vi "SetPeddleRate.vi"(8 "error in (no error)":errorcluster, 10 "peddle rate":dbl, 11 "Bike in":refnum<class "Bike.lvclass">) -> (0 "error out":errorcluster, 3 "Bike out":refnum<class "Bike.lvclass">)   [LabVIEW 2019, in "Bike.lvclass"]
uses:
  Bike.lvclass
  Bike.lvclass/Bike.ctl
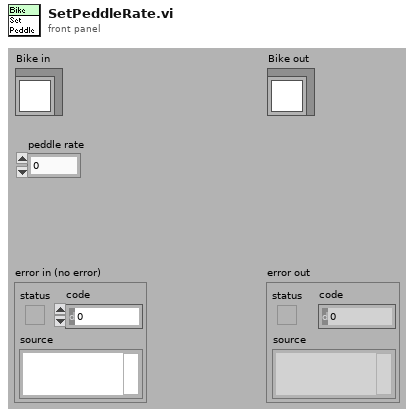
[diagram p1: front panel]
types:
  T1 = typedef "Bike.lvclass/DataRef.ctl" = refnum<data-value>
  T2 = typedef "Bike.lvclass/DataMembers.ctl" = cluster{"peddle rate":dbl}
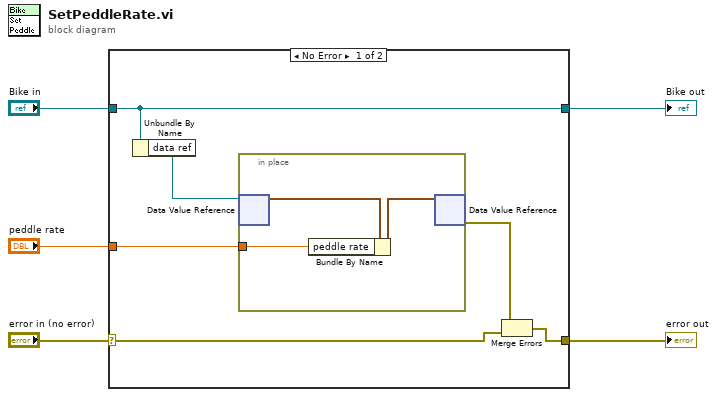
[diagram p0: block diagram]
diagram:
  n1 = case shown="No Error" "error in (no error)" {
    selector: "error in (no error)" -> [w7 w16]
    tunnel: [w6 w16] -> w4
    tunnel: [w11 w15] -> w2
    tunnel: "Bike in" -> [w11 w15]
    tunnel: "peddle rate" -> [w9 _]
    frame No Error {
      n2 = Unbundle By Name(w11) -> ("data ref"=w10:T1)
      n3 = in-place {
        in-place-border: w9 -> [w12]
        n4 = in-place-dvr #1(w10) -> (w14:T2)  [unwired: 1 out]
        n5 = Bundle By Name(cluster=w14, "peddle rate"=w12) -> (w13:T2)
        n6 = in-place-dvr #1(w13) -> (w8:errorcluster)  [unwired: 1 out]
      }
      n7 = Merge Errors(w8, w7) -> (w6:errorcluster)
    }
    frame Error {
    }
  }
  "error out" <- w4
  "Bike out" <- w2
